vi "create_SIM921_Data_header_units.vi"() -> (3 "String":string)   [LabVIEW 2019]
uses:
  Instrument_Setup.vi
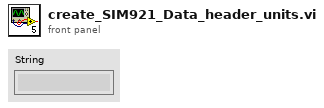
[diagram p1: front panel]
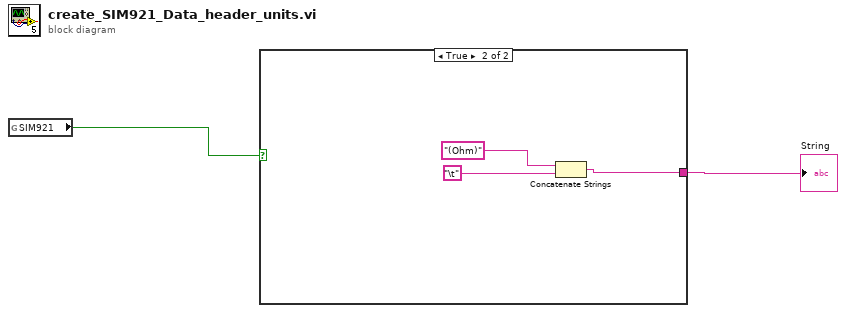
[diagram p0: block diagram]
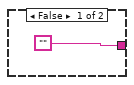
[diagram p2: hidden frame]
diagram:
  n1 = global read "Instrument_Setup.vi" "SIM921"() -> (w2:bool)
  n2 = case shown="True" w2 {
    tunnel: ["" w4] -> w1
    frame False {
    }
    frame True {
      n3 = Concatenate Strings("(Ohm)", "\t") -> (w4:string)
    }
  }
  "String" <- w1
